vi "SendMessage.vi"(7 "Message":string, 11 "error in (no error)":errorcluster) -> (0 "error out":errorcluster)   [LabVIEW 2020, in "ConsoleOutput.lvclass"]
uses:
  ConsoleOutput.lvclass
  Lib/hse-logger.lvlib
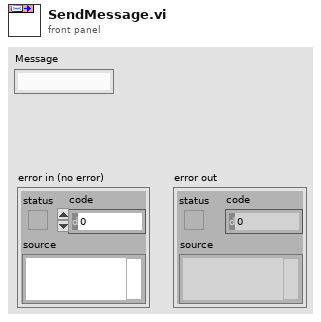
[diagram p1: front panel]
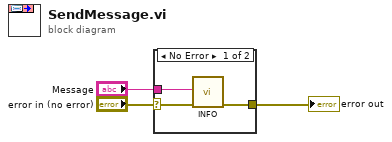
[diagram p0: block diagram]
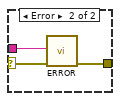
[diagram p2: hidden frame]
diagram:
  n1 = case shown="No Error" "error in (no error)" {
    selector: "error in (no error)" -> [w5 w9]
    tunnel: [w4 w8] -> w2
    tunnel: "Message" -> [w6 w7]
    frame No Error {
      n2 = call "INFO.vi"("Message"=w6, "error in"=w5) -> ("error out"=w4:errorcluster)  [unwired: 9 in]
    }
    frame Error {
      n3 = call "ERROR.vi"("Message"=w7, "error in"=w9) -> ("error out"=w8:errorcluster)  [unwired: 9 in]
    }
  }
  "error out" <- w2
